vi "Create PUBLISH msg.vi"(8 "error in":errorcluster, 10 "Publish Requst":T1, 11 "Request ID":u64) -> (0 "error out":errorcluster, 3 "WAMP Message":string)   [LabVIEW 2020, in "wamplv.lvlib" / "WAMP Client.lvclass"]
uses:
  WAMP Client.lvclass
  TypeDef/PUBLISH Request Data.ctl
  TypeDef/PUBLISH result.ctl
  API/TypeDefs/Combined error.ctl
  API/TypeDefs/WAMP error.ctl
  TypeDef/WAMP Message Codes.ctl
  <vilib>/JDP Science/JSONtext/JSONtext.lvlib
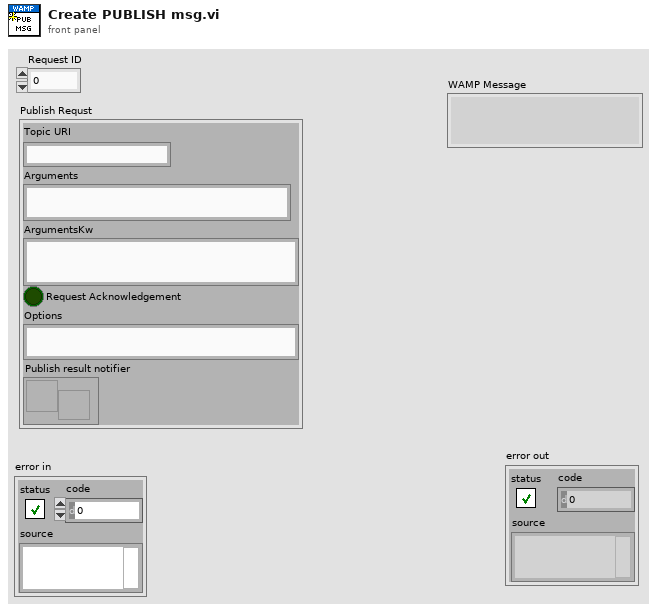
[diagram p1: front panel]
types:
  T1 = typedef "wamplv.lvlib/WAMP Client.lvclass/PUBLISH Request Data.ctl" = cluster{"Topic URI":string, "Arguments":string, "ArgumentsKw":string, "Request Acknowledgement":bool, "Options":string, "Publish result notifier":refnum<notifier>}
  T2 = typedef "wamplv.lvlib/WAMP Client.lvclass/WAMP Message Codes.ctl" = u16
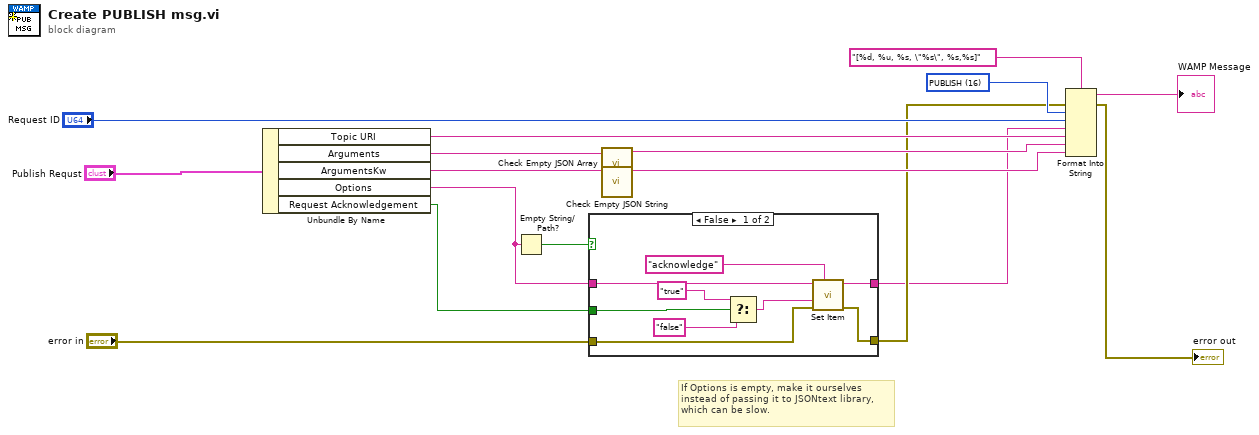
[diagram p0: block diagram]
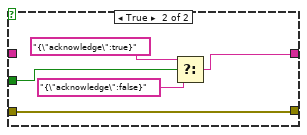
[diagram p2: hidden frame]
diagram:
  w15 = T2 16 items=["HELLO"=1, "WELCOME"=2, "ABORT"=3, "GOODBYE"=6, "ERROR"=8, "PUBLISH"=16, "PUBLISHED"=17, "SUBSCRIBE"=32, "SUBSCRIBED"=33, "UNSUBSCRIBE"=34, "UNSUBSCRIBED"=35, "EVENT"=36, "CALL"=48, "RESULT"=59, "REGISTER"=64, "REGISTERED"=65, "UNREGISTER"=66, "UNREGISTERED"=67, "INVOCATION"=68, "YIELD"=70] ("Message Codes")
  # "If Options is empty, make it ourselves \ninstead of passing it to JSONtext library, \nwhich can be slow."
  n1 = Unbundle By Name("Publish Requst") -> ("Topic URI"=w14:string, "Arguments"=w11:string, "ArgumentsKw"=w13:string, "Options"=w2:string, "Request Acknowledgement"=w1:bool)
  n2 = Empty String/Path?(string/path=w2) -> (empty?=w3:bool)
  n3 = case shown="False" w3 {
    tunnel: [w25 w29] -> w6
    tunnel: "error in" -> [w24 w29]
    tunnel: [w23 w28] -> w4
    tunnel: w2 -> [w22 _]
    tunnel: w1 -> [w18 w27]
    frame False {
      n4 = Select(t="true" ("JSON to Insert"), s=w18, f="false") -> (s? t:f=w19:string)
      n5 = call <vilib>:"Set Item.vi"("$Path or Item Name"="acknowledge", "error in (no error)"=w24, "JSON to Insert"=w19, "JSON"=w22) -> ("error out"=w25:errorcluster, "<JSON>"=w23:string)  [unwired: 4 in, 1 out]
    }
    frame True {
      n6 = Select(t="{\"acknowledge\":true}" ("JSON to Insert"), s=w27, f="{\"acknowledge\":false}") -> (s? t:f=w28:string)
    }
  }
  n7 = call "Check Empty JSON Array.vi"("JSON in"=w11) -> ("JSON out"=w10:string)  [unwired: 10 in]
  n8 = call "Check Empty JSON String.vi"("JSON in"=w13) -> ("JSON out"=w12:string)  [unwired: 10 in]
  n9 = Format Into String(format string="[%d, %u, %s, \"%s\", %s,%s]" ("element"), error in=w6, w15, "Request ID", w4, w14, w10, w12) -> (resulting string=→"WAMP Message":string, error out=→"error out":errorcluster)  [unwired: 1 in]
